vi "Right Level 2 Front Rocket.vi"() -> (4 "path":cluster{"X":dbl, "Y":dbl}[](array[cluster])=[{"X"=19.5, "Y"=112.0}, {"X"=20.500010188638996, "Y"=112.00000114918859}, {"X"=21.50000828269578, "Y"=111.99999382491393}, {"X"=22.499994643823822, "Y"=111.99998129735859}, {"X"=23.49997591045523, "Y"=111.99996889431097}, {"X"=24.499960594130847, "Y"=111.99996144150649}, {"X"=25.499954558599157, "Y"=111.99996132640938}, {"X"=26.499958715989486, "Y"=111.99996791746342}, {"X"=27.499969595425018, "Y"=111.99997831500777}, {"X"=28.49998187293667, "Y"=111.99998885197617}, {"X"=29.499991220781748, "Y"=111.99999658726765}, {"X"=30.499996059462948, "Y"=112.00000021151553}, {"X"=31.499997623298476, "Y"=112.00000014831821}, {"X"=32.49999865303651, "Y"=111.99999799183028}, {"X"=33.500001587960035, "Y"=111.99999563844496}, {"X"=34.50000718418369, "Y"=111.99999450149706}, {"X"=35.500014128670934, "Y"=111.99999507936361}, {"X"=36.50001969055315, "Y"=111.9999969592323}, {"X"=37.500021004971586, "Y"=111.99999916476611}, {"X"=38.500016381420124, "Y"=112.0000006531353}, {"X"=39.50000609944111, "Y"=112.00000075393118}, {"X"=40.499992419957294, "Y"=111.99999940319152}, {"X"=41.4999788659682, "Y"=111.99999712353953}, {"X"=42.49996908346738, "Y"=111.99999479613442}, {"X"=43.49996570395893, "Y"=111.99999333170894}, {"X"=44.49996958143441, "Y"=111.99999336349494}, {"X"=45.49997961235006, "Y"=111.99999505854785}, {"X"=46.4999931397696, "Y"=111.99999809209136}, {"X"=47.50000676504036, "Y"=112.00000177270012}, {"X"=48.50001729189343, "Y"=112.00000526243605}, {"X"=49.50002252499316, "Y"=112.00000781606313}, {"X"=50.50002172252699, "Y"=112.0000089688387}, {"X"=51.500015624653294, "Y"=112.00000862714116}, {"X"=52.500006104641365, "Y"=112.00000704995958}, {"X"=53.49999558245245, "Y"=112.00000474104064}, {"X"=54.49998638171956, "Y"=112.00000229279584}, {"X"=55.49998019852652, "Y"=112.00000022986131}, {"X"=56.49997779663298, "Y"=111.99999889305712}, {"X"=57.49997896980129, "Y"=111.99999838765876}, {"X"=58.49998273990558, "Y"=111.99999859943058}, {"X"=59.49998770715003, "Y"=111.99999926375122}, {"X"=60.49999244544543, "Y"=112.00000006171116}, {"X"=61.49999584234702, "Y"=112.00000071415582}, {"X"=62.499997312205736, "Y"=112.00000104963448}, {"X"=63.49999685237639, "Y"=112.00000103256863}, {"X"=64.49999495369002, "Y"=112.00000075020445}, {"X"=65.4999924082985, "Y"=112.0000003676869}, {"X"=66.49999007475442, "Y"=112.00000006743961}, {"X"=67.49998866060103, "Y"=111.99999999084481}, {"X"=68.49998856953921, "Y"=112.0000001973046}, {"X"=69.49998983866503, "Y"=112.00000064951173}, {"X"=70.49999216750496, "Y"=112.00000122615812}, {"X"=71.49999502015969, "Y"=112.00000175635707}, {"X"=72.49999776865238, "Y"=112.00000206531467}, {"X"=73.49999984118494, "Y"=112.0000020190716}, {"X"=74.50000084293715, "Y"=112.0000015574593}, {"X"=75.5000006271321, "Y"=112.00000070809344}, {"X"=76.49999930728445, "Y"=111.99999957914473}, {"X"=77.49999721467505, "Y"=111.99999833354646}, {"X"=78.49999481553292, "Y"=111.99999715114171}, {"X"=79.49999260850592, "Y"=111.99999618733663}, {"X"=80.49999102423921, "Y"=111.99999553687339}, {"X"=81.49999034575491, "Y"=111.99999520958202}, {"X"=82.49999066209487, "Y"=111.99999512196754}, {"X"=83.49999185997663, "Y"=111.99999510498178}, {"X"=84.49999365067843, "Y"=111.99999492505765}, {"X"=85.49999562333666, "Y"=111.99999431306357}, {"X"=86.49999731217936, "Y"=111.99999299461345}, {"X"=87.4999982642164, "Y"=111.99999071525335}, {"X"=88.49999809533234, "Y"=111.99998725524962}, {"X"=89.49999652597435, "Y"=111.99998243067208}, {"X"=90.49999339185803, "Y"=111.9999760797497}, {"X"=91.49998862946282, "Y"=111.9999680355932}, {"X"=92.49998223981027, "Y"=111.9999580879774}, {"X"=93.49997423657064, "Y"=111.999945937682}, {"X"=94.49996458568282, "Y"=111.99993114683808}, {"X"=95.49995314338878, "Y"=111.99991308786896}, {"X"=96.4999395981099, "Y"=111.99989089212053}, {"X"=97.49992341929014, "Y"=111.99986339740174}, {"X"=98.49990381362024, "Y"=111.99982909163448}, {"X"=99.4998796863396, "Y"=111.99978604787535}, {"X"=100.4998496029142, "Y"=111.99973184424353}, {"X"=101.49981174448617, "Y"=111.99966346083349}, {"X"=102.4997638491734, "Y"=111.99957714444021}, {"X"=103.49970313046353, "Y"=111.99946823074909}, {"X"=104.49962616345171, "Y"=111.99933091232705}, {"X"=105.49952872925081, "Y"=111.99915793903787}, {"X"=106.4994056072805, "Y"=111.99894023511072}, {"X"=107.49925030401998, "Y"=111.99866641371874}, {"X"=108.49905470491048, "Y"=111.9983221652704}, {"X"=109.49880863314793, "Y"=111.99788948937447}, {"X"=110.49849929490445, "Y"=111.99734573226709}, {"X"=111.49811058439387, "Y"=111.99666238102367}, {"X"=112.4976222183177, "Y"=111.99580355222054}, {"X"=113.49700863408907, "Y"=111.99472409971938}, {"X"=114.49623770695224, "Y"=111.99336722039298}, {"X"=115.49526879264708, "Y"=111.99166153708019}, {"X"=116.49405126480147, "Y"=111.98951711456219}, {"X"=117.49252050114812, "Y"=111.98682131181408}, {"X"=118.49059648335702, "Y"=111.98343178390446}, {"X"=119.48817756720587, "Y"=111.97917044241673}, {"X"=120.48513626879998, "Y"=111.97381284644742}, {"X"=121.48131270431566, "Y"=111.96707679917888}, {"X"=122.47650553125132, "Y"=111.9586079094983}, {"X"=123.4704615134564, "Y"=111.94796050549388}, {"X"=124.46286254141255, "Y"=111.934574061494}, {"X"=125.45330877716343, "Y"=111.91774398863807}, {"X"=126.44129739136919, "Y"=111.89658461524908}, {"X"=127.42619613473498, "Y"=111.86998237743327}, {"X"=128.40721021088424, "Y"=111.83653712395476}, {"X"=129.38334046666466, "Y"=111.79448853131001}, {"X"=130.3533307069768, "Y"=111.74162355231013}, {"X"=131.3156015111402, "Y"=111.67515990257996}, {"X"=132.2681671325842, "Y"=111.59159953249485}, {"X"=133.20853104720592, "Y"=111.48654449366846}, {"X"=134.13355457538032, "Y"=111.35446552129793}, {"X"=135.03929165420504, "Y"=111.1884110770488}, {"X"=135.92078110992492, "Y"=110.97964148056153}, {"X"=136.77178553703706, "Y"=110.71716888514032}, {"X"=137.61349179672317, "Y"=110.387178936069}, {"X"=138.44780001855833, "Y"=110.00348554306511}, {"X"=139.2762209816442, "Y"=109.5770761201182}, {"X"=140.0999556153901, "Y"=109.11668989676278}, {"X"=140.91995818811975, "Y"=108.62927787777387}, {"X"=141.73698652524058, "Y"=108.12036866446806}, {"X"=142.55164190313863, "Y"=107.5943594117934}, {"X"=143.36440070966842, "Y"=107.05474725137007}, {"X"=144.1756395262359, "Y"=106.50431336195362}, {"X"=144.98565494634497, "Y"=105.94526936385998}, {"X"=145.79467917672574, "Y"=105.3793737292376}, {"X"=146.60289224954178, "Y"=104.80802432973047}, {"X"=147.41043149438562, "Y"=104.2323319968455}, {"X"=148.21739876969218, "Y"=103.65317897576541}, {"X"=149.0238658308239, "Y"=103.07126535615124}, {"X"=149.82987811257877, "Y"=102.48714592457637}, {"X"=150.6354571221204, "Y"=101.90125937363733}, {"X"=151.44060156832123, "Y"=101.31395139880475}, {"X"=152.24528728904912, "Y"=100.7254928949827}, {"X"=153.04946597873945, "Y"=100.13609420754442}, {"X"=153.8530626309922, "Y"=99.54591621268447}, {"X"=154.65597165328577, "Y"=98.95507870292433}, {"X"=155.458051130508, "Y"=98.36366696707378}, {"X"=156.2591157618312, "Y"=97.77173551817481}, {"X"=157.0589264838513, "Y"=97.1793125886461}, {"X"=157.85717845588124, "Y"=96.58639903528268}, {"X"=158.6534849771656, "Y"=95.99297131254511}, {"X"=159.44735646096703, "Y"=95.3989782264168}, {"X"=160.2381754532273, "Y"=94.80433846780662}, {"X"=161.02516403877453, "Y"=94.20893722539282}, {"X"=161.80734239419684, "Y"=93.61261963771499}, {"X"=162.58347742744124, "Y"=93.01518225781122}, {"X"=163.35201820963866, "Y"=92.41636269626002}, {"X"=164.1110142058683, "Y"=91.81582605383097}, {"X"=164.85801235963277, "Y"=91.21314710110296}, {"X"=165.5899280275285, "Y"=90.60778770063257}, {"X"=166.30288283167874, "Y"=89.99906855658348}, {"X"=166.99200058532685, "Y"=89.38613362417826}, {"X"=167.65115052506584, "Y"=88.7679050753149}, {"X"=168.27262453319284, "Y"=88.14302646571365}, {"X"=168.84673148161153, "Y"=87.50979126786163}, {"X"=169.3612872785457, "Y"=86.86605308365654}, {"X"=169.8009736506131, "Y"=86.20911275313388}, {"X"=170.14653187323387, "Y"=85.53557632850104}, {"X"=170.37374907789166, "Y"=84.84117641524308}, {"X"=170.48498887264287, "Y"=84.09642214312304}, {"X"=170.50398426300046, "Y"=83.31161791935483}, {"X"=170.44961331269835, "Y"=82.49496023944397}, {"X"=170.33689274815933, "Y"=81.65296911528797}, {"X"=170.17776829021454, "Y"=80.7908312489956}, {"X"=169.98174333495726, "Y"=79.91267300507728}, {"X"=169.75637910739792, "Y"=79.02177756282484}, {"X"=169.50769262755782, "Y"=78.12075769929228}, {"X"=169.2404734235744, "Y"=77.21169330694717}, {"X"=168.95853563704497, "Y"=76.2962408780643}, {"X"=168.66491877218985, "Y"=75.37572070430144}, {"X"=168.36204765456174, "Y"=74.45118637024622}, {"X"=168.05186003172685, "Y"=73.52348019748528}, {"X"=167.73590854723355, "Y"=72.59327756449778}, {"X"=167.41544246208278, "Y"=71.66112244404557}, {"X"=167.09147342080666, "Y"=70.72745603333091}, {"X"=166.7648287129436, "Y"=69.7926399826465}, {"X"=166.43619482336103, "Y"=68.85697543761232}, {"X"=166.10615355878892, "Y"=67.9207189042962}, {"X"=165.77521267294563, "Y"=66.9840957096554}, {"X"=165.44383249853595, "Y"=66.04731198238343}, {"X"=165.11245047609356, "Y"=65.11056519452514}, {"X"=164.7815033358877, "Y"=64.17405507613553}, {"X"=164.45145178893762, "Y"=63.23799349736052}, {"X"=164.1228023536745, "Y"=62.30261603849987}, {"X"=163.79613625839823, "Y"=61.36819444681511}, {"X"=163.472139181518, "Y"=60.43505058867742}, {"X"=163.15163666076975, "Y"=59.5035735587308}, {"X"=162.83563837706967, "Y"=58.57424033408455}, {"X"=162.52539144140545, "Y"=57.64764072121795}, {"X"=162.22244546440848, "Y"=56.72450828218852}, {"X"=161.9287340341126, "Y"=55.80575904422388}, {"X"=161.64667686579358, "Y"=54.89253981078644}, {"X"=161.37930729053156, "Y"=53.98628847389663}, {"X"=161.1304316772623, "Y"=53.08880960641866}, {"X"=160.90482958866946, "Y"=52.20236943879238}, {"X"=160.70850542187074, "Y"=51.32981519962414}, {"X"=160.54900460303216, "Y"=50.474725006949505}, {"X"=160.43581074933286, "Y"=49.64159616238102}, {"X"=160.38084469554747, "Y"=48.83608180259899}, {"X"=160.39909180391746, "Y"=48.06528841848294}, {"X"=160.5093906792067, "Y"=47.33814990774086}, {"X"=160.7354247652864, "Y"=46.66589781362905}, {"X"=161.100002537277, "Y"=46.04336377430019}, {"X"=161.57477665560174, "Y"=45.460375780074}, {"X"=162.13719958856564, "Y"=44.908843179234914}, {"X"=162.7693368491195, "Y"=44.38233084739258}, {"X"=163.4569230760857, "Y"=43.875720508495256}, {"X"=164.18861126735257, "Y"=43.38494136892681}, {"X"=164.9553756096864, "Y"=42.90675587275072}, {"X"=165.75003644397796, "Y"=42.43858929757798}, {"X"=166.56688236405682, "Y"=41.97839422933461}, {"X"=167.40136958341841, "Y"=41.524542793878844}, {"X"=168.24988277233817, "Y"=41.07574097975096}, {"X"=169.10954478652008, "Y"=40.6309605410649}, {"X"=169.9780652626811, "Y"=40.18938488952013}, {"X"=170.85362009353824, "Y"=39.75036612118133}, {"X"=171.7347554288196, "Y"=39.31339091251118}, {"X"=172.62031112811528, "Y"=38.87805350331528}, {"X"=173.50935975451773, "Y"=38.44403429963746}, {"X"=174.40115749217094, "Y"=38.01108316852425}, {"X"=175.2951056834362, "Y"=37.5790059603279}, {"X"=176.19071792834507, "Y"=37.14765493545125}, {"X"=177.0875966399869, "Y"=36.71692002738401}, {"X"=177.9854098445608, "Y"=36.28672406985108}, {"X"=178.8838751143235, "Y"=35.857018125879016}, {"X"=179.78274470868865, "Y"=35.42777888009337}, {"X"=180.6817917606915, "Y"=34.99900776734969}, {"X"=181.58079870566925, "Y"=34.57073082881489}, {"X"=182.47954601850645, "Y"=34.143000162469484}, {"X"=183.37780059563224, "Y"=33.715896337424645}, {"X"=184.27530333181795, "Y"=33.28953325561151}, {"X"=185.17175527328612, "Y"=32.864063679833215}, {"X"=186.06680241663466, "Y"=32.43968734708083}, {"X"=186.96001698130627, "Y"=32.01666161218833}, {"X"=187.85087454517387, "Y"=31.59531487233048}, {"X"=188.73872655360964, "Y"=31.17606386813727}, {"X"=189.6227663687765, "Y"=30.759435700786014}, {"X"=190.50198674349343, "Y"=30.34609552779294}, {"X"=191.37512671225667, "Y"=29.93688150110207}, {"X"=192.24060527357412, "Y"=29.532848911234872}, {"X"=193.09643824245092, "Y"=29.135325794764608}, {"X"=193.94013378603483, "Y"=28.7459828327951}, {"X"=194.79478592474507, "Y"=28.35445707391347}, {"X"=195.65728569531592, "Y"=27.961528238931447}, {"X"=196.5249371984853, "Y"=27.56790218763719}, {"X"=197.39531572787658, "Y"=27.174248096210825}, {"X"=198.26614010930348, "Y"=26.78123368152357}, {"X"=199.13515258817506, "Y"=26.38956032978717}, {"X"=200.0, "Y"=26.0}])   [LabVIEW 2018]
uses:
  AutonBuilder/Typedef/Data Point.ctl
panel:
  in  "Data Points":T1[](array[typedef])=[{"X"=19.5, "Y"=112.0, "Theta"=0.0, "Speed %"=0.0, "Disabled?"=FALSE}, {"X"=136.94845360824743, "Y"=112.0, "Theta"=0.0, "Speed %"=0.0, "Disabled?"=FALSE}, {"X"=172.57731958762886, "Y"=85.79790940766551, "Theta"=0.0, "Speed %"=0.0, "Disabled?"=FALSE}, {"X"=158.10309278350516, "Y"=45.721254355400696, "Theta"=0.0, "Speed %"=0.0, "Disabled?"=FALSE}, {"X"=193.7319587628866, "Y"=28.787456445993033, "Theta"=0.0, "Speed %"=0.0, "Disabled?"=FALSE}, {"X"=200.0, "Y"=26.0, "Theta"=0.0, "Speed %"=0.0, "Disabled?"=FALSE}]
  out "Graph":cluster{dbl[], dbl[]}[](graph)=[{[0.0, 33.5, 33.5, 0.0, 0.0], [126.25, 126.25, 97.75, 97.75, 126.25]}, {[19.5, 136.94845360824743, 172.57731958762886, 158.10309278350516, 193.7319587628866, 200.0], [112.0, 112.0, 85.79790940766551, 45.721254355400696, 28.787456445993033, 26.0]}, {array[254 elements], array[254 elements]}, {array[254 elements], array[254 elements]}, {array[254 elements], array[254 elements]}]
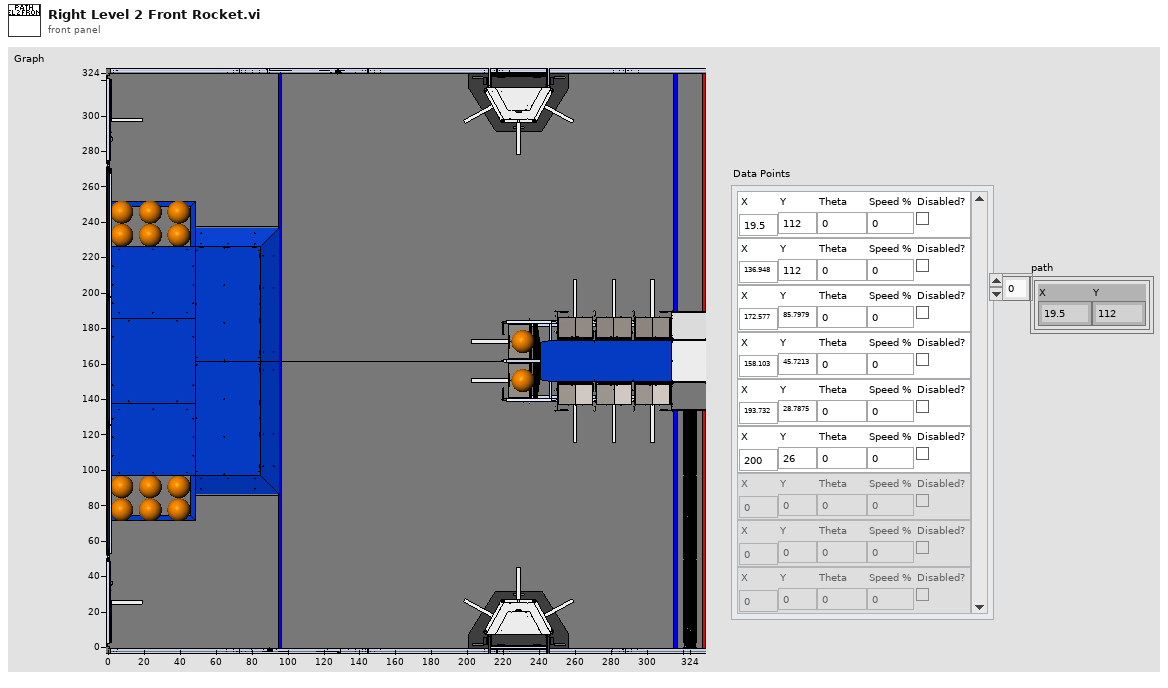
[diagram p1: front panel]
types:
  T1 = typedef "Data Point.ctl" = cluster{"X":dbl, "Y":dbl, "Theta":dbl, "Speed %":dbl, "Disabled?":bool}
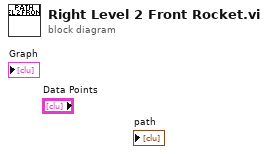
[diagram p0: block diagram]
diagram:
